vi "ProcessMetaData.vi"(1 "Number of Lines (1)":i32=1, 2 "Header":string, 3 "MetaData":string) -> (0 "Data":string)   [LabVIEW 2016, in "ExpData.lvclass"]
uses:
  ExpData.lvclass
  <vilib>/AuZn/auzn custom VIs/AuZnCustomVI.lvlib
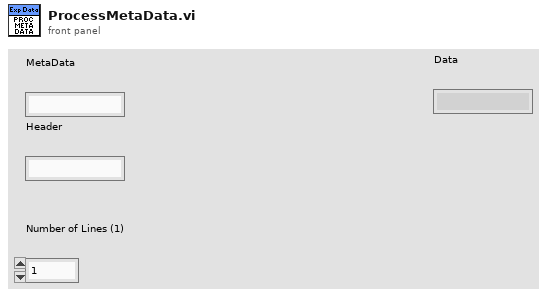
[diagram p1: front panel]
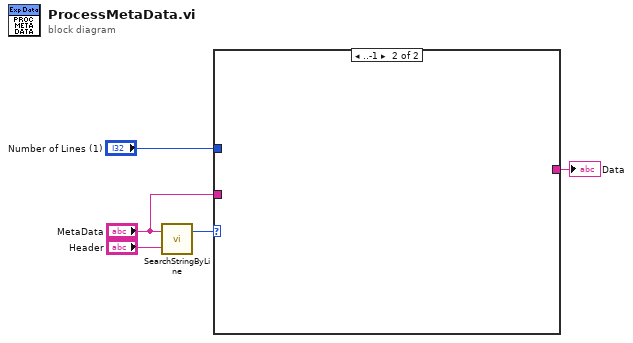
[diagram p0: block diagram]
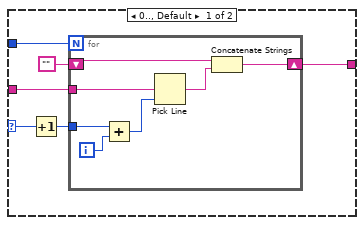
[diagram p2: hidden frame]
diagram:
  n1 = call <vilib>:"SearchStringByLine.vi"("String"="Header", "Input Multi-line String"="MetaData") -> ("Line Number"=w4:i32)  [unwired: 1 in]
  n2 = case shown="..-1" w4 {
    selector: w4 -> [w11 _]
    tunnel: "Number of Lines (1)" -> [w9 _]
    tunnel: "MetaData" -> [w8 _]
    tunnel: [w7 _] -> w1
    frame 0.., Default {
      n3 = Increment(x=w11) -> (x+1=w10:i32)
      n4 = for {
        N: w9 -> [_]
        tunnel: w8 -> [w15]
        tunnel: w10 -> [w17]
        shift-right: [w12] -> w7
        shift-left: "" -> [w14]
        i -> [w18]
        n5 = Add(x=w17, y=w18) -> (x+y=w16:i32)
        n6 = Pick Line(multi-line string=w15, line index=w16) -> (output string=w13:string)  [unwired: 1 in]
        n7 = Concatenate Strings(w14, w13) -> (w12:string)
      }
    }
    frame ..-1 {
    }
  }
  "Data" <- w1
